vi "receiveTEDSStatus.vi"(8 "error in (no error)":errorcluster, 11 "ILC in":refnum<class "ILC.lvclass">) -> (0 "error out":errorcluster, 2 "TEDS Status":string, 3 "ILC out":refnum<class "ILC.lvclass">)   [LabVIEW 2015, in "ILCCommon.lvlib" / "ILC.lvclass"]
uses:
  <userlib>/Common/ILC/ILC/ILC.lvclass
  <userlib>/Common/ILC/ILCModelTypedefs/FinalDelimiter.ctl
  <userlib>/Common/ILC/ILCModelTypedefs/ILCModelTypedefs.lvlib
  <userlib>/Common/SerialProtocols/SerialCommunicator/SerialCommunicator.lvclass
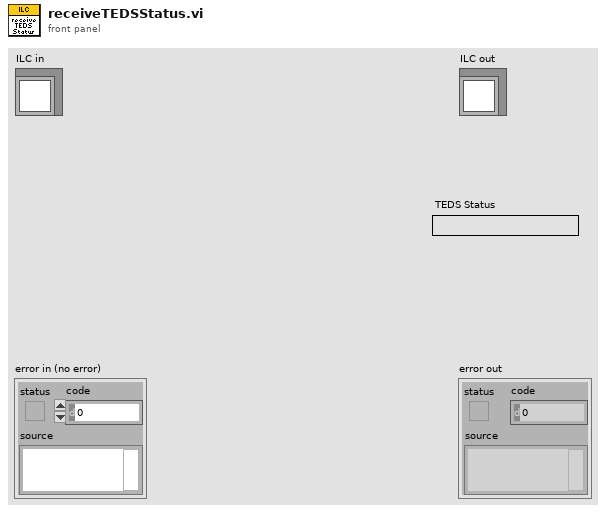
[diagram p1: front panel]
types:
  T1 = typedef "ILCCommon.lvlib/ILCModelTypedefs.lvlib/FinalDelimiter.ctl" = enum16{",", "<CR><LF>"}
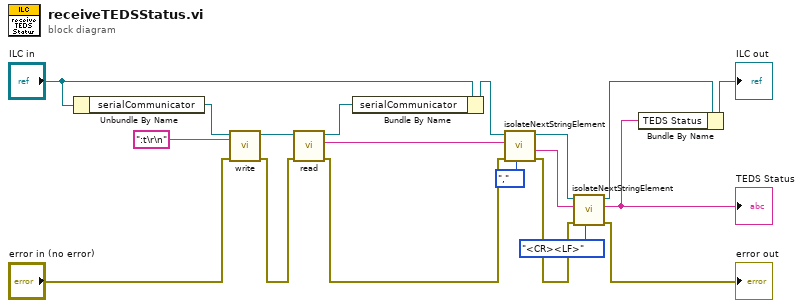
[diagram p0: block diagram]
diagram:
  n1 = Unbundle By Name("ILC in") -> ("serialCommunicator"=w13:refnum<class "SerialCommunicator.lvclass">)
  n2 = call-dynamic "write.vi"("error in (no error)"="error in (no error)", "writeString"=":t\r\n", "SerialCommunicator in"=w13) -> ("error out"=w3:errorcluster, "SerialCommunicator out"=w15:refnum<class "SerialCommunicator.lvclass">)  [unwired: 7 in]
  n3 = call-dynamic "read.vi"("error in (no error)"=w3, "SerialCommunicator in"=w15) -> ("error out"=w2:errorcluster, "stringRead"=w8:string, "SerialCommunicator out"=w6:refnum<class "SerialCommunicator.lvclass">)  [unwired: 7 in]
  n4 = Bundle By Name(cluster="ILC in", "serialCommunicator"=w6) -> (w5:refnum<class "ILC.lvclass">)
  n5 = call <userlib>:"isolateNextStringElement.vi"("Final Delimiter"=FinalDelimiter.",", "error in (no error)"=w2, "inputString"=w8, "ILC in"=w5) -> ("error out"=w1:errorcluster, "remainingString"=w18:string, "ILC out"=w17:refnum<class "ILC.lvclass">)  [unwired: 4 in, 1 out]
  n6 = call <userlib>:"isolateNextStringElement.vi"("Final Delimiter"=FinalDelimiter."<CR><LF>", "error in (no error)"=w1, "inputString"=w18, "ILC in"=w17) -> ("error out"=→"error out":errorcluster, "extractedSegment"=w10:string, "ILC out"=w4:refnum<class "ILC.lvclass">)  [unwired: 4 in, 1 out]
  "TEDS Status" <- w10
  n7 = Bundle By Name(cluster=w4, "TEDS Status"=w10) -> (→"ILC out":refnum<class "ILC.lvclass">)
